vi "TDMS - Playback Control.vi"() -> ()   [LabVIEW 2011]
doc: "Sample numeric display item."
uses:
  <vilib>/NI Veristand/Display Template Support/Display Template Support.llb/cluster_Screen Item Settings.ctl
  <vilib>/NI Veristand/Display Template Support/Display Template Support.llb/cluster_Graph Scale Settings.ctl
  <vilib>/NI Veristand/Display Template Support/Display Template Support.llb/cluster_Graph Plot Settings.ctl
  <vilib>/NI Veristand/Display Template Support/Display Template Support.llb/enum_Display Template Handler Minimal To Widget Msg.ctl
  <vilib>/NI Veristand/Display Template Support/Display Template Support.llb/enum_Display Template Handler Minimal To Workspace.ctl
  <vilib>/regexp/Match Regular Expression.xnode
  <vilib>/NI Veristand/Execution/Workspace/NI_VS Workspace ExecutionAPI.lvlib
panel:
  in  "NIVS.Gateway IP Address":string
  in  "Selector":T1(ring)=enum."Loop"
  in  "Item.Data":T2
  out "Label":string="TDMS Control"
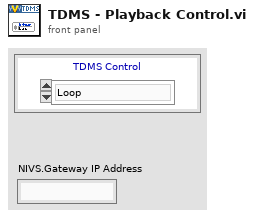
[diagram p1: front panel]
types:
  T1 = enum16{"Play and Repeat Last", "Stop (and Reset)", "Loop", "Pause"}
  T2 = typedef "cluster_Screen Item Settings.ctl" = cluster{"Template VI":string, "Position X":i32, "Position Y":i32, "Custom":string, "Show Title Bar":bool, "ID":i32, "Always On Top":bool, "Allow Resize":bool, "Allow Minimize":bool, "Allow Close":bool, "Size to Screen":bool, "Screen.ID":i32, "State":enum16{"Normal", "New"}, "Title":string, "Window Bounds":cluster{"[0]":i16, "[1]":i16, "[2]":i16, "[3]":i16}, "Channel Ref":u64, "Unit":string, "Default Units?":bool, "Flash Limit?":bool, "Color 1":u32, "Color 2":u32, "Color 3":u32, "Color 4":u32, "Bck Color":u32, "Fore Color":u32, "Limit 1":dbl, "Limit 2":dbl, "Limit 3":dbl, "Limit 4":dbl, "Limit Mode 1":i32, "Limit Mode 2":i32, "Limit Mode 3":i32, "Limit Mode 4":i32, "Scale Precision":i32, "Scale Min":dbl, "Scale Max":dbl, "Format":i32, "Precision":i32, "Background Type":i32, "IDs":i32[], "Units":string[], "Labels":string[], "Scale Factor":dbl, "Scale Offset":dbl, "YScale Index":u32[], "XScale":T3, "YScales":T3[], "Plots":T4[], "Update Period":dbl, "History Length":dbl, "My.Ref":refnum<vi>, "Is Control?":bool, "Channel Paths":string[], "Custom Data":variant}
  T3 = typedef "cluster_Graph Scale Settings.ctl" = cluster{"Format":u8, "Precision":u8, "Fit":u8, "Label":string, "Use Default Label":bool, "Label Visible":bool, "Min":dbl, "Max":dbl}
  T4 = typedef "cluster_Graph Plot Settings.ctl" = cluster{"Bar Style":u8, "Fill To":i16, "Fill/PtColor":u32, "Line Style":u8, "Line Width":u8, "Color":u32, "Interp":u8, "Point Style":u8}
  T5 = typedef "enum_Display Template Handler Minimal To Workspace.ctl" = cluster{"Operation":enum16{"SetCustomData", "DeleteItem"}, "Data":variant}
  T6 = typedef "enum_Display Template Handler Minimal To Widget Msg.ctl" = enum16{"Stop", "LaunchConfigDialog"}
  T7 = typedef "NI_VS Workspace ExecutionAPI.lvlib/WorkspaceAPI.ctl" = refnum<k24>
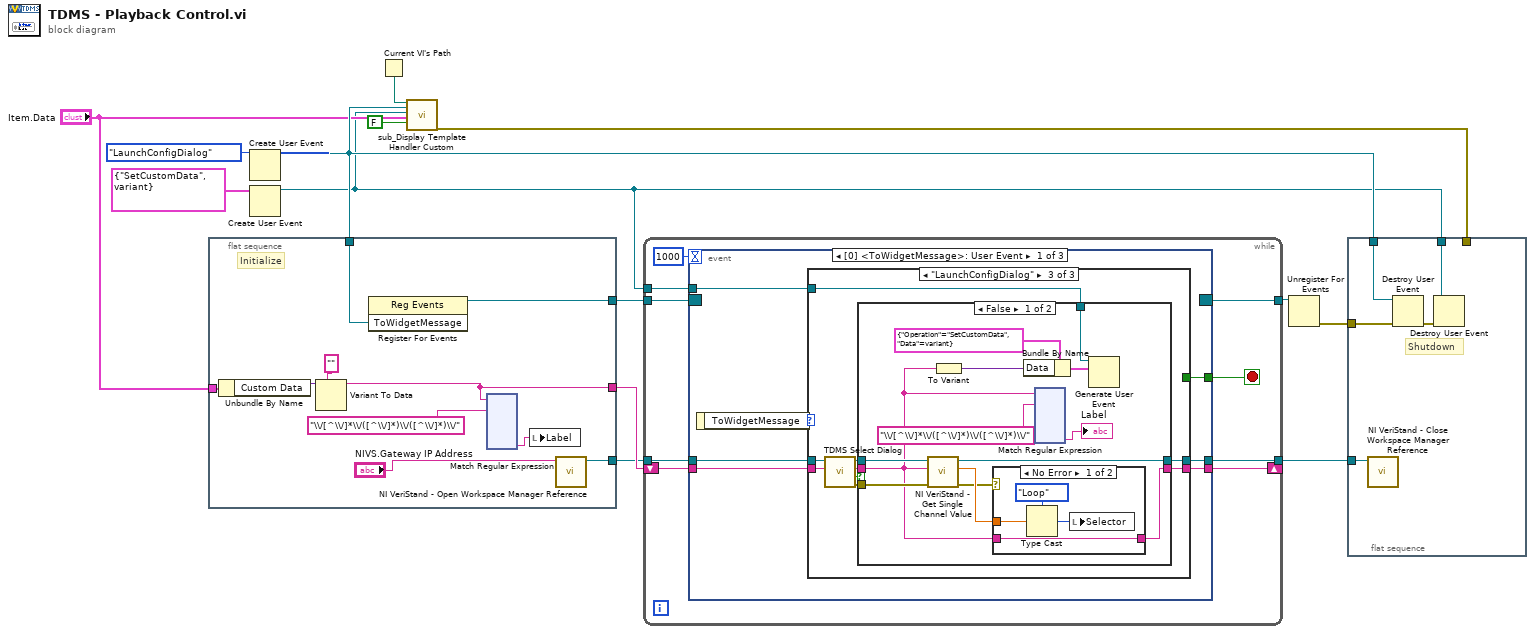
[diagram p0: block diagram]
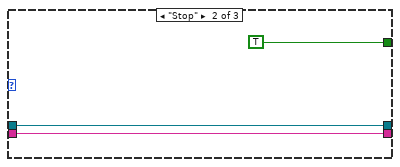
[diagram p3: hidden frame]
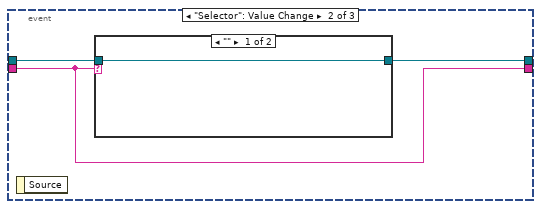
[diagram p6: hidden frame]
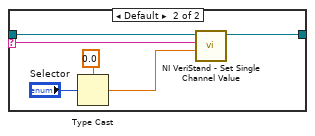
[diagram p7: hidden frame]
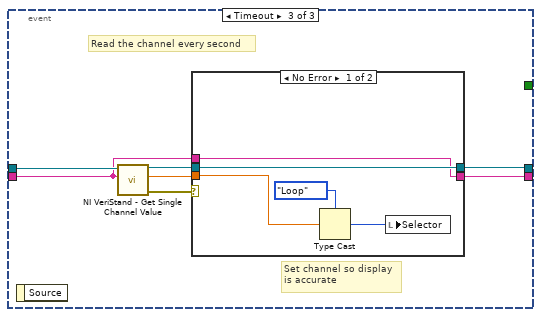
[diagram p8: hidden frame]
diagram:
  n1 = flat-sequence {
    tunnel: [w24] -> w12
    tunnel: w9 -> [w23]
    tunnel: "Item.Data" -> [w22]
    tunnel: [w17] -> w3
    tunnel: [w18] -> w2
    frame #0 {
      # "Initialize"
      n2 = Unbundle By Name(w22) -> ("Custom Data"=w21:variant)
      n3 = Variant To Data(type="" ("Channel"), Variant=w21) -> (data=w17:string)  [unwired: 1 in, 1 out]
      n4 = register-events(w23) -> (reference out=w24:refnum<event-registration>)  [unwired: 2 in, 1 out]
      n5 = xnode "Match Regular Expression"("input string"=w17, "regular expression"="\\/[^\\/]*\\/([^\\/]*)\\/([^\\/]*)\\/") -> ("submatch 2"=w15:string)  [unwired: 2 in, 8 out]
      n6 = local write "Label"(w15) -> ()
      n7 = call <vilib>:"NI VeriStand - Open Workspace Manager Reference.vi"("Gateway IP Address (\"\": localhost)"="NIVS.Gateway IP Address") -> ("WorkspaceManager"=w18:T7)  [unwired: 1 in, 9 out]
    }
  }
  n8 = Create User Event(user event datatype=enum_Display_Template_Handler_Minimal_To_Widget_Msg."LaunchConfigDialog" ("ToWidgetMessage")) -> (user event=w9:refnum<user-event>)  [unwired: 1 in, 1 out]
  n9 = Create User Event(user event datatype=T5 {"Operation"=enum."SetCustomData", "Data"=variant} ("Data")) -> (user event=w5:refnum<user-event>)  [unwired: 1 in, 1 out]
  n10 = Current VI's Path() -> (path=w7:path)
  n11 = call <vilib>:"sub_Display Template Handler Custom.vi"("Parent.Path"=w7, "ToWidgetEvent"=w9, "ToWorkspace"=w5, "Item.Data"="Item.Data", "Resizable"=FALSE) -> ("error out"=w14:errorcluster)  [unwired: 14 in]
  n12 = while {
    tunnel: w12 -> [w147]
    tunnel: [w145] -> w11
    tunnel: w5 -> [w144]
    tunnel: w2 -> [w142]
    tunnel: [w141] -> w1
    shift-right: [w140] -> _
    shift-left: w3 -> [w143]
    stop <- w146 stop-if-true
    n13 = event shown="[0] <ToWidgetMessage>: User Event" {
      selector: w147 -> [_ _ _]
      dyn-events: [_ _ _] -> w145
      timeout: 1000 -> [_ _ _]
      tunnel: [w153 _ _] -> w146
      tunnel: w144 -> [w152 _ _]
      tunnel: w143 -> [w149 w303 w313]
      tunnel: w142 -> [w151 w305 w319]
      tunnel: [w148 w304 w318] -> w141
      tunnel: [w150 w303 w314] -> w140
      event User Event {
        n14 = event-data() -> ("ToWidgetMessage"=w154:T6)  [unwired: 1 out]
        n15 = case shown="\"LaunchConfigDialog\"" w154 {
          tunnel: [_ TRUE _] -> w153
          tunnel: w152 -> [_ _ w168]
          tunnel: w151 -> [w155 w157 w167]
          tunnel: [w156 w158 w160] -> w150
          tunnel: w149 -> [w156 w158 w165]
          tunnel: [w155 w157 w161] -> w148
          frame Default {
          }
          frame "Stop" {
          }
          frame "LaunchConfigDialog" {
            n16 = call "TDMS Select Dialog.vi"("Node"=w165, "WorkspaceManager"=w167) -> ("error out"=w164:errorcluster, "Cancelled?"=w166:bool, "Channel"=w162:string, "WorkspaceManager out"=w163:T7)  [unwired: 1 in, 5 out]
            n17 = case shown="False" w166 {
              tunnel: w168 -> [w181 _]
              tunnel: w164 -> [w175 _]
              tunnel: w163 -> [w176 w302]
              tunnel: w162 -> [w171 w301]
              tunnel: [w173 w302] -> w161
              tunnel: [w170 w301] -> w160
              frame False {
                n18 = call <vilib>:"NI VeriStand - Get Single Channel Value.vi"("error in (no error)"=w175, "Channel"=w171, "WorkspaceManager in"=w176) -> ("error out"=w172:errorcluster, "Value"=w174:dbl, "WorkspaceManager out"=w173:T7)  [unwired: 6 in]
                n19 = To Variant(anything=w171) -> (Variant=w178:variant)
                n20 = case shown="No Error" w172 {
                  tunnel: w174 -> [w184 _]
                  tunnel: w171 -> [w182 w186]
                  tunnel: [w182 w186] -> w170
                  frame No Error {
                    n21 = Type Cast(type=T1."Loop" ("Selector"), x=w184) -> (*(type *) &x=w185:T1)
                    n22 = local write "Selector"(w185) -> ()
                  }
                  frame Error {
                  }
                }
                n23 = Bundle By Name(cluster=T5 {"Operation"=enum."SetCustomData", "Data"=variant} ("event data"), "Data"=w178) -> (w179:T5)
                n24 = xnode "Match Regular Expression"("input string"=w171, "regular expression"="\\/[^\\/]*\\/([^\\/]*)\\/([^\\/]*)\\/") -> ("submatch 2"=→"Label":string)  [unwired: 2 in, 8 out]
                n25 = Generate User Event(user event=w181, event data cluster=w179) -> ()  [unwired: 1 in, 2 out]
              }
              frame True {
              }
            }
          }
        }
      }
      event "Selector": Value Change {
        n26 = event-data() -> ()  [unwired: 2 out]
        n27 = case shown="\"\"" w303 {
          selector: w303 -> [_ w307]
          tunnel: w305 -> [w306 w312]
          tunnel: [w306 w308] -> w304
          frame "" {
          }
          frame Default {
            n28 = Type Cast(type=0.0, x="Selector") -> (*(type *) &x=w310:dbl)
            n29 = call <vilib>:"NI VeriStand - Set Single Channel Value.vi"("Value"=w310, "Channel"=w307, "WorkspaceManager in"=w312) -> ("WorkspaceManager out"=w308:T7)  [unwired: 7 in, 1 out]
          }
        }
      }
      event Timeout {
        # "Read the channel every second"
        # "Set channel so display\nis accurate"
        n30 = event-data() -> ()  [unwired: 2 out]
        n31 = call <vilib>:"NI VeriStand - Get Single Channel Value.vi"("Channel"=w313, "WorkspaceManager in"=w319) -> ("error out"=w315:errorcluster, "Value"=w316:dbl, "WorkspaceManager out"=w317:T7)  [unwired: 7 in]
        n32 = case shown="No Error" w315 {
          tunnel: w316 -> [w324 _]
          tunnel: [w321 w326] -> w318
          tunnel: w317 -> [w321 w326]
          tunnel: [w320 w325] -> w314
          tunnel: w313 -> [w320 w325]
          frame No Error {
            n33 = Type Cast(type=T1."Loop" ("Selector"), x=w324) -> (*(type *) &x=w322:T1)
            n34 = local write "Selector"(w322) -> ()
          }
          frame Error {
          }
        }
      }
    }
  }
  n35 = Unregister For Events(event registration refnum=w11) -> (error out=w10:errorcluster)  [unwired: 1 in]
  n36 = flat-sequence {
    tunnel: w14 -> [_]
    tunnel: w10 -> [w330]
    tunnel: w9 -> [w331]
    tunnel: w5 -> [w328]
    tunnel: w1 -> [w327]
    frame #0 {
      # "Shutdown"
      n37 = call <vilib>:"NI VeriStand - Close Workspace Manager Reference.vi"("WorkspaceManager"=w327) -> ()  [unwired: 1 in, 10 out]
      n38 = Destroy User Event(user event=w331, error in=w330) -> (error out=w329:errorcluster)
      n39 = Destroy User Event(user event=w328, error in=w329) -> ()  [unwired: 1 out]
    }
  }
